vi "Raw Data to Waveform.vi"(8 "error in (no error)":errorcluster, 9 "I32 data":i32[][](array[numeric]), 10 "I16 data":i16[][](array[numeric]), 11 "Pulse Driver in":refnum<class "Pulse Driver.lvclass">) -> (0 "error out":errorcluster, 2 "Array":waveform(dbl)[](array[waveform]), 3 "Pulse Driver out":refnum<class "Pulse Driver.lvclass">)   [LabVIEW 2020, in "Pulse Driver.lvclass"]
uses:
  Pulse Driver.lvclass
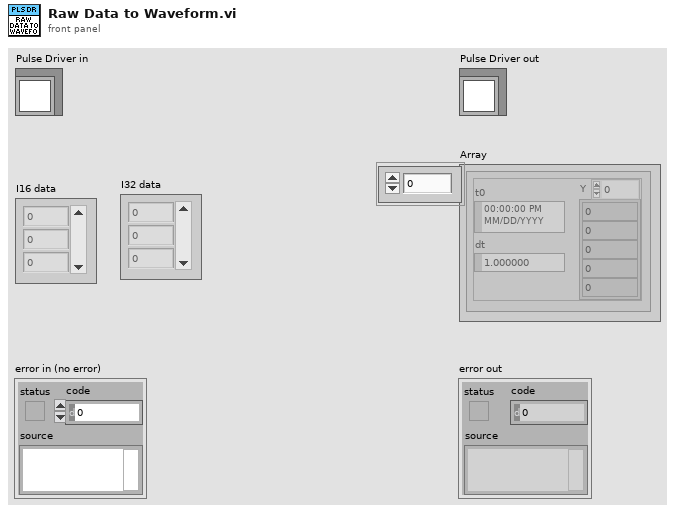
[diagram p1: front panel]
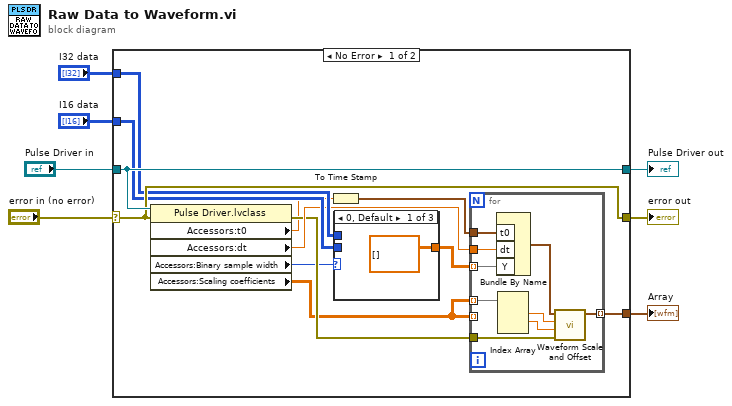
[diagram p0: block diagram]
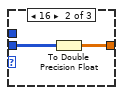
[diagram p2: hidden frame]
diagram:
  n1 = case shown="No Error" "error in (no error)" {
    selector: "error in (no error)" -> [w18 w34]
    tunnel: [w18 w34] -> w6
    tunnel: [w19 w33] -> w4
    tunnel: "Pulse Driver in" -> [w19 w33]
    tunnel: "I16 data" -> [w17 _]
    tunnel: "I32 data" -> [w16 _]
    tunnel: [w10 _] -> w1
    frame No Error {
      n2 = property class="Pulse Driver.lvclass"(reference=w19, error in=w18) -> (error out=w12:errorcluster, "Accessors:t0"=w9:dbl, "Accessors:dt"=w13:dbl, "Accessors:Binary sample width"=w8:i32, "Accessors:Scaling coefficients"=w11:dbl[][])  [unwired: 1 out]
      n3 = To Time Stamp(1:w9) -> (0:w14:timestamp)
      n4 = case shown="0, Default" w8 {
        tunnel: w17 -> [_ w31 _]
        tunnel: [dbl[][] [] ("I32 data") w30 w32] -> w15
        tunnel: w16 -> [_ _ w32]
        frame 0, Default {
        }
        frame 16 {
          n5 = To Double Precision Float(number=w31) -> (double precision float=w30:dbl[][])
        }
        frame 32 {
        }
      }
      n6 = for {
        tunnel: w15 -> [w26] mode=indexing
        tunnel: w14 -> [w28]
        tunnel: w13 -> [w27]
        tunnel: w11 -> [_] mode=indexing
        tunnel: w12 -> [w24]
        tunnel: w11 -> [w23] mode=indexing
        tunnel: [w20] -> w10 mode=indexing
        n7 = Bundle By Name("t0"=w28, "dt"=w27, "Y"=w26) -> (w25:waveform(dbl))  [unwired: 1 in]
        n8 = Index Array(array=w23) -> (element #1=w22:dbl, element #2=w21:dbl)  [unwired: 3 in, 1 out]
        n9 = call <vilib>:"Waveform Scale and Offset.vi"("error in (no error)"=w24, "scale"=w21, "offset"=w22, "waveform in"=w25) -> ("waveform out"=w20:waveform(dbl))  [unwired: 6 in, 1 out]
      }
    }
    frame Error {
    }
  }
  "error out" <- w6
  "Pulse Driver out" <- w4
  "Array" <- w1
